vi "Loop.vi"(9 "Error Queue":refnum<queue>, 10 "Event Actor Queue":refnum<queue>, 11 "jettl Event Actor in":refnum<class "jettl Event Actor.lvclass">) -> ()   [LabVIEW 2021, in "jettl.lvlib" / "jettl Event Actor.lvlib" / "jettl Event Actor.lvclass"]
uses:
  jettl Event Actor.lvclass
  Actor/Event Actor/Event Actor.lvclass
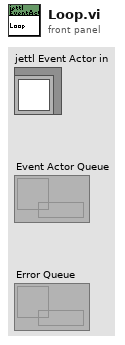
[diagram p1: front panel]
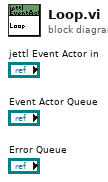
[diagram p0: block diagram]
diagram:
